vi "Parse Config File.vi"(8 "error in (no error)":errorcluster, 10 "Section":string, 11 "Config Path":path) -> (0 "error out":errorcluster, 3 "Array":T1[](array[typedef]))   [LabVIEW 2022 SP3, in "Read Configs Sections.lvlib"]
uses:
  Read Configs Sections.lvlib
  Section Data.ctl
  <vilib>/Utility/config.llb/Read Key (String).vi
  <vilib>/Utility/error.llb/Error Cluster From Error Code.vi
  <vilib>/Utility/config.llb/Read Key (Path).vi
  <vilib>/ErrorRing/Error Ring.xnode
  <vilib>/Utility/config.llb/NI_LVConfig.lvlib
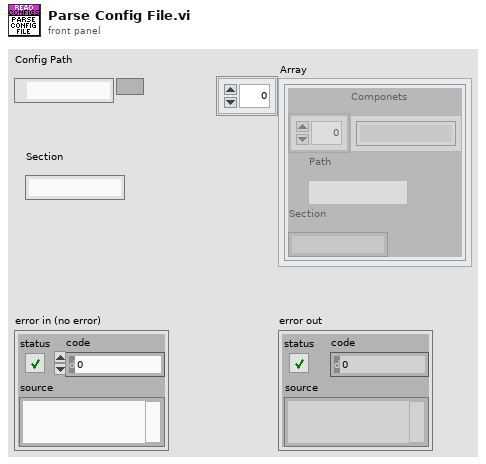
[diagram p1: front panel]
types:
  T1 = typedef "Read Configs Sections.lvlib/Section Data.ctl" = cluster{"Componets":string[], "Path":path, "Section":string}
  T2 = typedef "NI_LVConfig.lvlib/Config Data RefNum.ctl" = refnum<k1>
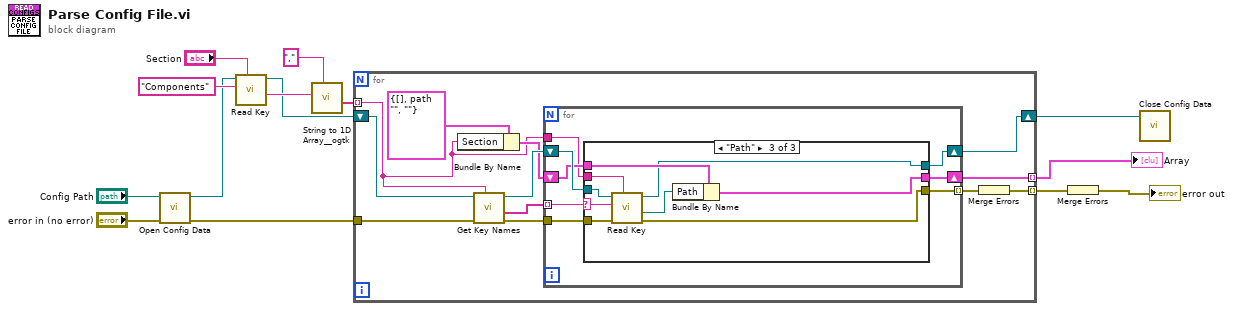
[diagram p0: block diagram]
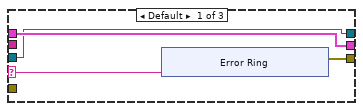
[diagram p2: hidden frame]
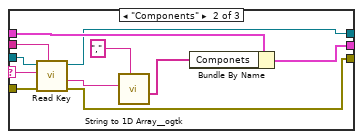
[diagram p3: hidden frame]
diagram:
  n1 = call <vilib>:"Open Config Data.vi"("error in (no error)"="error in (no error)", "configuration file path"="Config Path") -> ("error out"=w7:errorcluster, "refnum"=w3:T2)  [unwired: 7 in, 1 out]
  n2 = call-poly <vilib>:"Read Key.vi"("section"="Section", "key"="Components", "refnum"=w3) -> ("value"=w5:string, "refnum out"=w2:T2)  [unwired: 5 in, 2 out]
  n3 = call <userlib>:"String to 1D Array__ogtk.vi"("delimiter (Tab)"=",", "string"=w5) -> ("Array of Strings"=w4:string[])  [unwired: 9 in]
  n4 = for {
    tunnel: [w23] -> w13 mode=indexing
    shift-right: [w21] -> w1
    shift-left: w2 -> [w26]
    tunnel: w7 -> [w19]
    tunnel: [w16] -> w10 mode=indexing
    tunnel: w4 -> [w15] mode=indexing
    n5 = Bundle By Name(cluster=T1 {"Componets"=[], "Path"=path "", "Section"=""} ("Cluster"), "Section"=w15) -> (w22:T1)
    n6 = call <vilib>:"Get Key Names.vi"("section"=w15, "error in (no error)"=w19, "refnum"=w26) -> ("error out"=w18:errorcluster, "key names"=w25:string[], "refnum out"=w24:T2)  [unwired: 5 in, 1 out]
    n7 = for {
      tunnel: w25 -> [w31] mode=indexing
      tunnel: w15 -> [w30]
      shift-right: [w33] -> w23
      shift-left: w22 -> [w32]
      shift-right: [w29] -> w21
      shift-left: w24 -> [w34]
      tunnel: w18 -> [w28]
      tunnel: [w27] -> w17 mode=indexing
      n8 = case shown="\"Path\"" w31 {
        selector: w31 -> [w37 w55 w64]
        tunnel: w34 -> [w36 w56 w65]
        tunnel: [w38 w54 w59] -> w33
        tunnel: w32 -> [w38 w53 w62]
        tunnel: w30 -> [_ w48 w63]
        tunnel: [w36 w49 w60] -> w29
        tunnel: w28 -> [_ w47 w58]
        tunnel: [w35 w46 w57] -> w27
        frame Default {
          n9 = xnode "Error Ring"("parameter 0"=w37) -> ("error out"=w35:errorcluster)
        }
        frame "Components" {
          n10 = call-poly <vilib>:"Read Key.vi"("section"=w48, "error in (no error)"=w47, "key"=w55, "refnum"=w56) -> ("error out"=w46:errorcluster, "value"=w52:string, "refnum out"=w49:T2)  [unwired: 4 in, 1 out]
          n11 = call <userlib>:"String to 1D Array__ogtk.vi"("delimiter (Tab)"=",", "string"=w52) -> ("Array of Strings"=w51:string[])  [unwired: 9 in]
          n12 = Bundle By Name(cluster=w53, "Componets"=w51) -> (w54:T1)
        }
        frame "Path" {
          n13 = call-poly <vilib>:"Read Key.vi"("section"=w63, "error in (no error)"=w58, "key"=w64, "refnum"=w65) -> ("error out"=w57:errorcluster, "value"=w61:path, "refnum out"=w60:T2)  [unwired: 4 in, 1 out]
          n14 = Bundle By Name(cluster=w62, "Path"=w61) -> (w59:T1)
        }
      }
    }
    n15 = Merge Errors(w17) -> (w16:errorcluster)
  }
  "Array" <- w13
  n16 = Merge Errors(w10) -> (→"error out":errorcluster)
  n17 = call <vilib>:"Close Config Data.vi"("refnum"=w1) -> ()  [unwired: 9 in, 2 out]
